vi "POST.vi"(0 "url":string, 1 "timeout_ms":i32, 2 "response_len_out":i32, 5 "headers_json":string, 7 "body_ptr":string, 9 "body_len":i32, 11 "error in (no error)":errorcluster, 12 "handle_out":cluster{}, 13 "status_out":u32) -> (4 "response_len_out out":i32, 6 "status_out out":u32, 8 "function return":i32, 14 "handle_out out":cluster{}, 15 "error out":errorcluster)   [LabVIEW 2020, in "reqwest-labview.lvlib"]
doc: "Performs an HTTP POST request with a raw binary body and returns a handle and response length for use with http_read_response.\n\n\n\n\n\nint http_post(const char *url,\n const char *headers_json,\n const unsigned char *body_ptr,\n int body_len,\n int timeout_ms,\n unsigned long long *handle_out,\n int *response_len_out,\n unsigned int *status_out);"
uses:
  reqwest-labview.lvlib
  http_rs_labview.dll
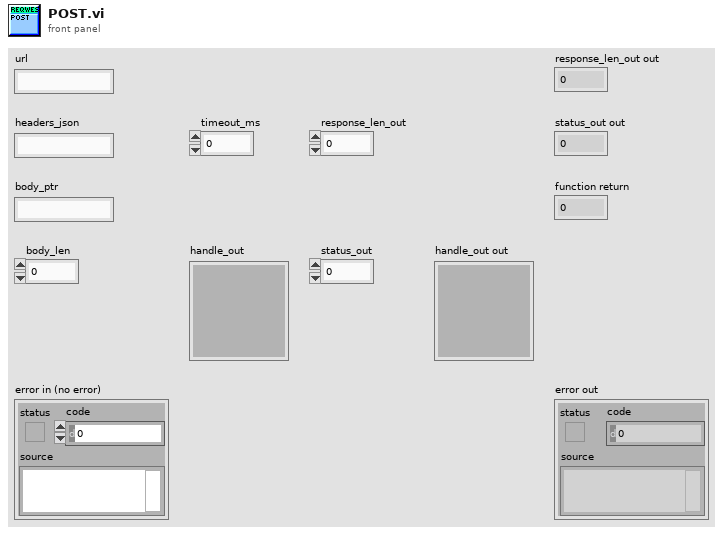
[diagram p1: front panel]
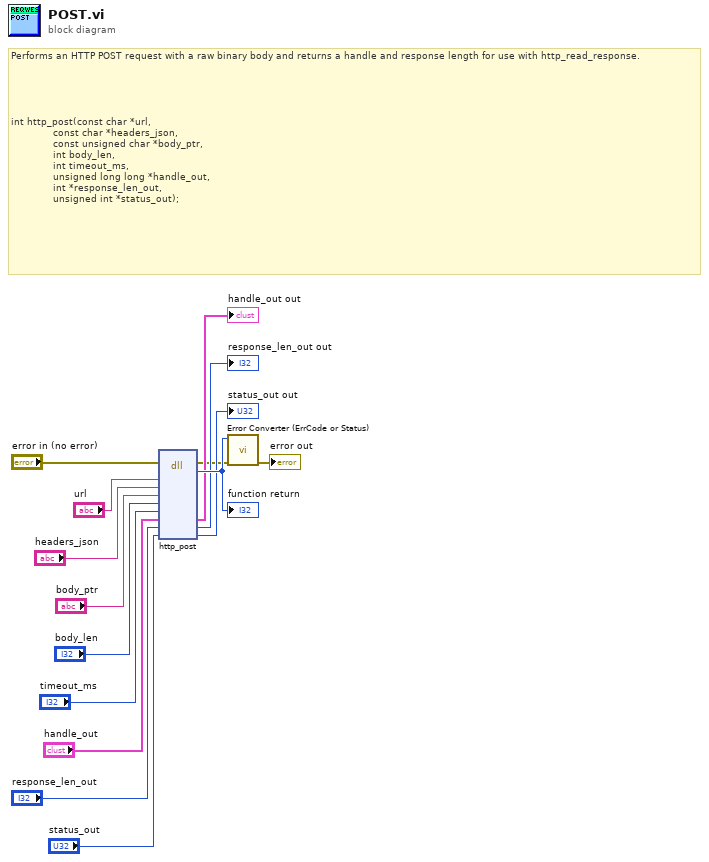
[diagram p0: block diagram]
diagram:
  # "Performs an HTTP POST request with a raw binary body and returns a handle and response length for use with http_read_response.\n\n\n\n\n\nint http_post(const char *url,\n              const char *headers_json,\n              const unsigned char *body_ptr,\n              int body_len,\n              int timeout_ms,\n              unsigned long long *handle_out,\n              int *response_len_out,\n              unsigned int *status_out);"
  n1 = dll-call lib="C:/code/reqwest-labview/lv-src/shared-library/http_rs_labview.*" fn="http_post"(error in="error in (no error)", "url"="url", "headers_json"="headers_json", "body_ptr"="body_ptr", "body_len"="body_len", "timeout_ms"="timeout_ms", "handle_out"="handle_out", "response_len_out"="response_len_out", "status_out"="status_out") -> (error out=w2:errorcluster, w15:i32, "handle_out"=→"handle_out out":cluster{}, "response_len_out"=→"response_len_out out":i32, "status_out"=→"status_out out":u32)  [unwired: 7 in, 1 out]
  "function return" <- w15
  n2 = call "Error Converter (ErrCode or Status).vi"("error in (no error)"=w2, "error code"=w15) -> ("error out"=→"error out":errorcluster)  [unwired: 9 in]
